vi "CallDAQReceiver.vi"(8 "error in":errorcluster) -> (0 "error out":errorcluster)   [LabVIEW 2014]
panel:
  # "Call DAQ Receiver"
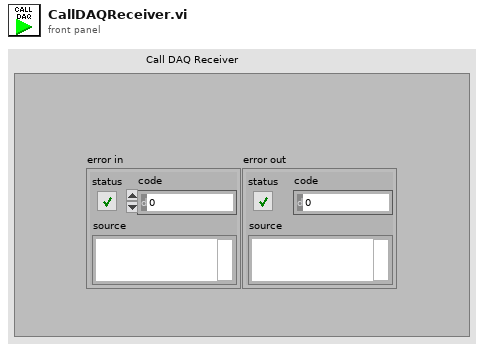
[diagram p1: front panel]
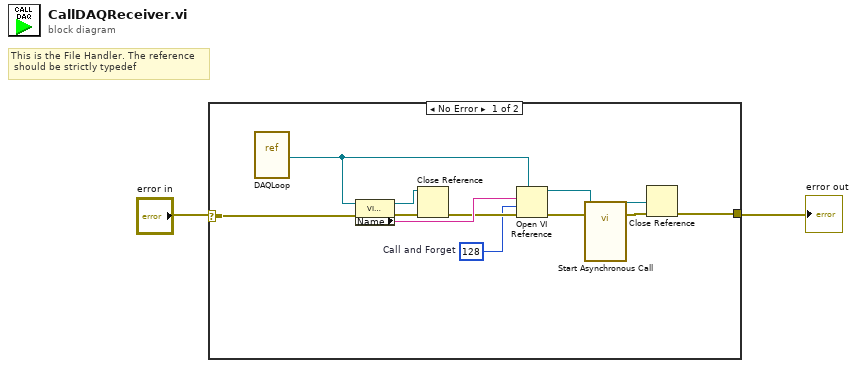
[diagram p0: block diagram]
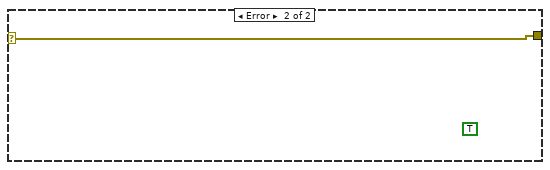
[diagram p2: hidden frame]
diagram:
  # "This is the File Handler. The reference\n should be strictly typedef"
  n1 = case shown="No Error" "error in" {
    selector: "error in" -> [w13 w15]
    tunnel: [w10 w15] -> w1
    frame No Error {
      w4 = 128  # Call and Forget
      n2 = vi-ref "DAQLoop.vi"() -> (w3:refnum<vi>)
      n3 = property class="VI (strict)"(reference=w3, error in=w13) -> (reference out=w5:refnum<vi>, error out=w7:errorcluster, "Name"=w8:string)
      n4 = Close Reference(reference=w5, error in (no error)=w7) -> (error out=w6:errorcluster)
      n5 = Open VI Reference(type specifier VI Refnum (for type only)=w3, vi path=w8, options=w4, error in (no error)=w6) -> (vi reference=w12:refnum<vi>, error out=w14:errorcluster)  [unwired: 2 in]
      n6 = call-by-ref "Start Asynchronous Call"(reference=w12, error in=w14) -> (reference out=w11:refnum<vi>, error out=w9:errorcluster)  [unwired: 12 in]
      n7 = Close Reference(reference=w11, error in (no error)=w9) -> (error out=w10:errorcluster)
    }
    frame Error {
      (unwired) TRUE
    }
  }
  "error out" <- w1
